vi "scan_DO_perform_scan.vi"(8 "error in (no error)":errorcluster, 10 "scan_settings":T1={"Center Pos. (mm)"=0.0, "Range [--|--]"=0.0, "Unit"=enum."mm", "Steps"=0.0, "Stage Number"=enum."1", "Stage Speed"=1.0, "Dwell Time (s)"=0.1, "Record Type"=enum."hdf5", "Save Path"=path "", "Notes"=""}, 11 "scan_panel in":refnum<class "scan_panel.lvclass">) -> (0 "error out":errorcluster, 3 "scan_panel out":refnum<class "scan_panel.lvclass">)   [LabVIEW 2015, in "scan_panel.lvclass"]
uses:
  scan_panel.lvclass
  scan_settings.ctl
  scan_unit.ctl
  scan_record.ctl
  scan_position_settings.ctl
  UI/front_panel_class/hardware_caller_queue_numbers.ctl
  Stage Class/Stage.lvclass
  Detector_Class/detector/detector.lvclass
  scan_hdf5_log/initialization_data.ctl
  scan_hdf5_log/scan_hdf5_log.lvclass
  Data Logger Class/data_logger.lvclass
  UI/panel_class/panel.lvclass
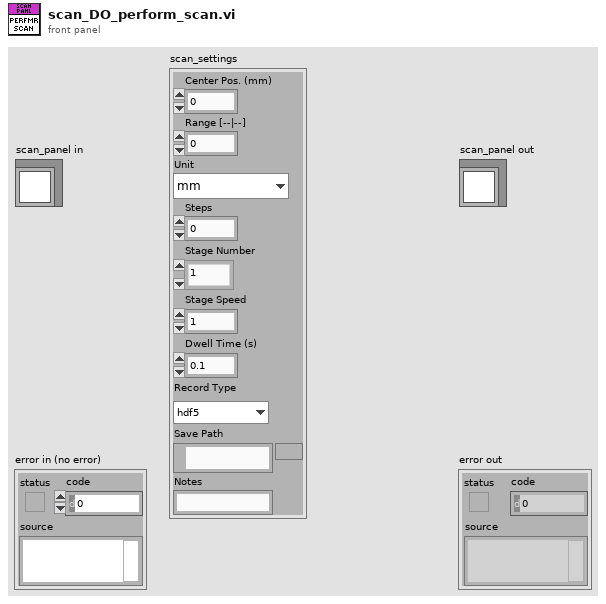
[diagram p1: front panel]
types:
  T1 = typedef "scan_settings.ctl" = cluster{"Center Pos. (mm)":dbl, "Range [--|--]":dbl, "Unit":T2, "Steps":dbl, "Stage Number":enum16{"1", "2"}, "Stage Speed":dbl, "Dwell Time (s)":dbl, "Record Type":T3, "Save Path":path, "Notes":string}
  T2 = typedef "scan_unit.ctl" = enum16{"mm", "s", "ms", "us", "ns", "ps", "fs"}
  T3 = typedef "scan_record.ctl" = enum16{"hdf5", "legacy", "None"}
  T4 = typedef "scan_position_settings.ctl" = cluster{"Center Pos. (mm)":dbl, "Range [--|--]":dbl, "Unit":T2, "Steps":dbl}
  T5 = typedef "initialization_data.ctl" = cluster{"Positions (mm)":dbl[], "dims":u32[]}
  T6 = typedef "hardware_caller_queue_numbers.ctl" = enum16{"stage1", "stage2", "experiment", "detector"}
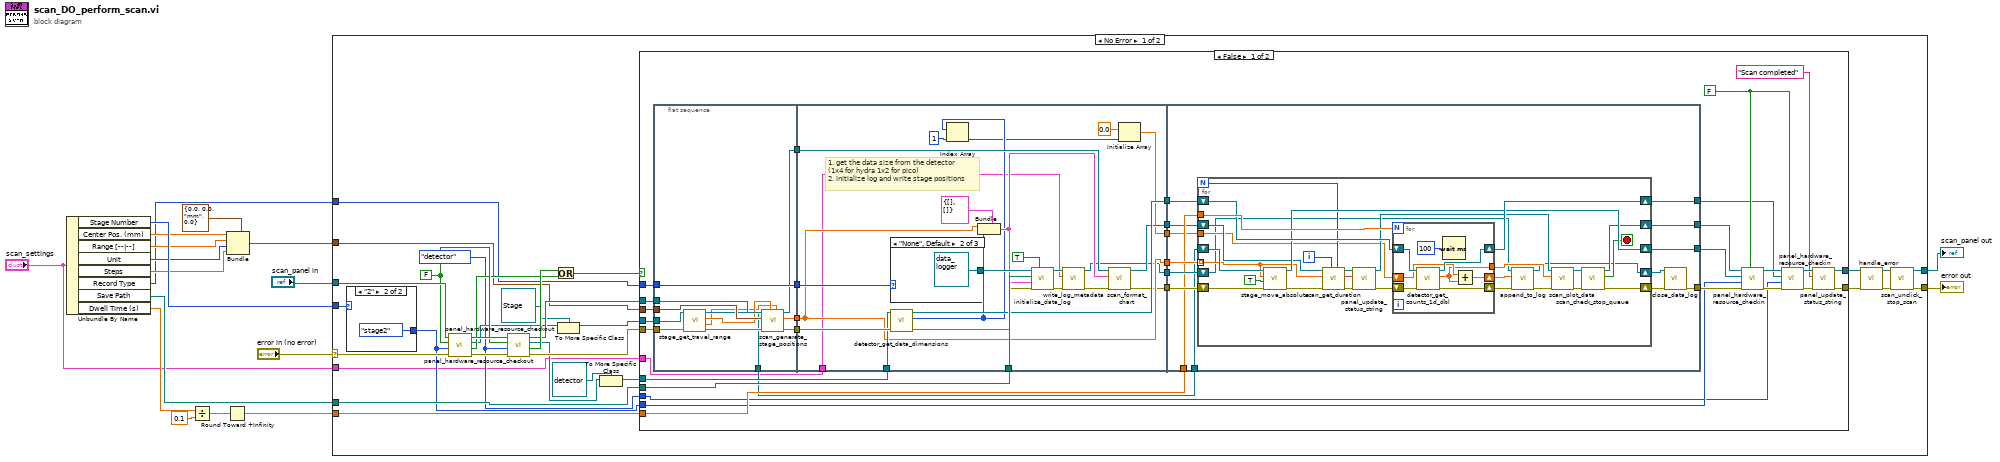
[diagram p0: block diagram]
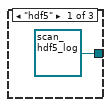
[diagram p2: hidden frame]
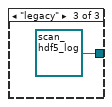
[diagram p3: hidden frame]
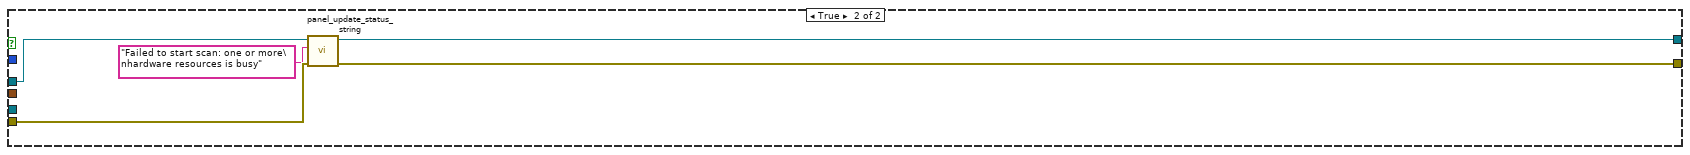
[diagram p4: hidden frame]
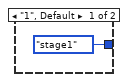
[diagram p5: hidden frame]
diagram:
  n1 = Unbundle By Name("scan_settings") -> ("Stage Number"=w14:enum16{"1", "2"}, "Center Pos. (mm)"=w13:dbl, "Range [--|--]"=w12:dbl, "Unit"=w11:T2, "Steps"=w10:dbl, "Record Type"=w7:T3, "Save Path"=w6:path, "Dwell Time (s)"=w5:dbl)
  n2 = Divide(x=w5, y=0.1) -> (x/y=w3:dbl)
  n3 = Round Toward +Infinity(x=w3) -> (ceil(x): smallest int >= x=w2:dbl)
  n4 = Bundle(cluster=T4 {"Center Pos. (mm)"=0.0, "Range [--|--]"=0.0, "Unit"=enum."mm", "Steps"=0.0} ("output cluster"), "Center Pos. (mm)"=w13, "Range [--|--]"=w12, "Unit"=w11, "Steps"=w10) -> (w8:T4)
  n5 = case shown="No Error" "error in (no error)" {
    selector: "error in (no error)" -> [w48 w181]
    tunnel: [w20 w181] -> w17
    tunnel: [w21 w180] -> w15
    tunnel: "scan_panel in" -> [w46 w180]
    tunnel: w14 -> [w47 _]
    tunnel: w8 -> [w37 _]
    tunnel: w7 -> [w36 _]
    tunnel: w6 -> [w35 _]
    tunnel: w2 -> [w28 _]
    tunnel: "scan_settings" -> [w19 _]
    frame No Error {
      w26 = hardware_caller_queue_numbers."detector" ("panel_number")
      w43 = FALSE ("Self?")
      n6 = case shown="\"2\"" w47 {
        tunnel: [hardware_caller_queue_numbers."stage1" ("panel_number") hardware_caller_queue_numbers."stage2" ("panel_number")] -> w27
        frame "1", Default {
        }
        frame "2" {
        }
      }
      n7 = call "panel_hardware_resource_checkout.vi"("error in (no error)"=w48, "panel_number"=w27, "Self?"=w43, "panel in"=w46) -> ("error out"=w45:errorcluster, "timed out?"=w41:bool, "hardware.lvclass"=w34:refnum<class "hardware.lvclass">, "panel out"=w44:refnum<class "scan_panel.lvclass">)  [unwired: 4 in]
      n8 = call "panel_hardware_resource_checkout.vi"("error in (no error)"=w45, "panel_number"=w26, "Self?"=w43, "panel in"=w44) -> ("error out"=w39:errorcluster, "timed out?"=w42:bool, "hardware.lvclass"=w31:refnum<class "hardware.lvclass">, "panel out"=w38:refnum<class "scan_panel.lvclass">)  [unwired: 4 in]
      n9 = Or(x=w42, y=w41) -> (x .or. y?=w40:bool)
      n10 = To More Specific Class(target class=refnum<class "Stage.lvclass"> refnum ("Stage.lvclass"), reference=w34) -> (specific class reference=w32:refnum<class "Stage.lvclass">)  [unwired: 1 in, 1 out]
      n11 = To More Specific Class(target class=refnum<class "detector.lvclass"> refnum ("detector.lvclass"), reference=w31) -> (specific class reference=w29:refnum<class "detector.lvclass">)  [unwired: 1 in, 1 out]
      n12 = case shown="False" w40 {
        tunnel: w39 -> [w79 w177]
        tunnel: w38 -> [w78 w175]
        tunnel: [w54 w174] -> w24
        tunnel: [w56 w176] -> w25
        tunnel: w37 -> [w77 _]
        tunnel: w36 -> [w75 _]
        tunnel: w35 -> [w73 _]
        tunnel: w32 -> [w51 _]
        tunnel: w29 -> [w70 _]
        tunnel: w28 -> [w64 _]
        tunnel: w27 -> [w61 _]
        tunnel: w26 -> [w59 _]
        tunnel: w19 -> [w49 _]
        frame False {
          w80 = FALSE ("Self")
          n13 = flat-sequence {
            tunnel: w79 -> [w88]
            tunnel: w78 -> [w94]
            tunnel: w77 -> [w93]
            tunnel: [w92] -> w76
            tunnel: w75 -> [w92]
            tunnel: [w91] -> w74
            tunnel: [w90] -> w72
            tunnel: [w89] -> w71
            tunnel: w51 -> [w86]
            tunnel: [w85] -> w50
            tunnel: w76 -> [w118]
            tunnel: w74 -> [w114]
            tunnel: w73 -> [w116]
            tunnel: w72 -> [w107]
            tunnel: w71 -> [w109]
            tunnel: w70 -> [w113]
            tunnel: [w106] -> w69
            tunnel: [w110] -> w68
            tunnel: [w97] -> w67
            tunnel: [w109] -> w66
            tunnel: [w108] -> w65
            tunnel: [w100] -> w52
            tunnel: w49 -> [w95]
            tunnel: w69 -> [w129]
            tunnel: w68 -> [w132]
            tunnel: w67 -> [w133]
            tunnel: w66 -> [w135]
            tunnel: w65 -> [w134]
            tunnel: w50 -> [w131]
            tunnel: w64 -> [w130]
            tunnel: [w126] -> w63
            tunnel: [w125] -> w62
            tunnel: [w124] -> w60
            tunnel: [w123] -> w58
            tunnel: w52 -> [w122]
            frame #0 {
              n14 = call-dynamic "stage_get_travel_range.vi"("error in (no error)"=w88, "Stage in"=w86) -> ("error out"=w87:errorcluster, "min(mm)"=w83:dbl, "max (mm)"=w84:dbl, "Stage out"=w85:refnum<class "Stage.lvclass">)  [unwired: 6 in]
              n15 = call "scan_generate_stage_positions.vi"("travel_min (mm)"=w83, "travel_max (mm)"=w84, "error in (no error)"=w87, "scan_position_settings"=w93, "scan_panel in"=w94) -> ("error out"=w91:errorcluster, "Positions (mm)"=w89:dbl[], "scan_panel out"=w90:refnum<class "scan_panel.lvclass">)  [unwired: 4 in]
            }
            frame #1 {
              # "1. get the data size from the detector \n(1x4 for hydra 1x2 for pico)\n2. initialize log and write stage positions"
              n16 = case shown="\"None\", Default" w118 {
                tunnel: [refnum<class "scan_hdf5_log.lvclass"> refnum ("scan_hdf5_log.lvclass") refnum<class "data_logger.lvclass"> refnum ("data_logger.lvclass") refnum<class "scan_hdf5_log.lvclass"> refnum ("scan_hdf5_log.lvclass")] -> w117
                frame "hdf5" {
                }
                frame "None", Default {
                }
                frame "legacy" {
                }
              }
              n17 = call-dynamic "detector_get_data_dimensions.vi"("error in (no error)"=w114, "detector in"=w113) -> ("error out"=w111:errorcluster, "dims"=w103:u32[], "detector out"=w110:refnum<class "detector.lvclass">)  [unwired: 6 in, 1 out]
              n18 = Index Array(array=w103, index=1) -> (element=w101:u32)
              n19 = Bundle(cluster=T5 {"Positions (mm)"=[], "dims"=[]} ("output cluster"), "Positions (mm)"=w109, "dims"=w103) -> (w105:T5)
              n20 = call-dynamic "initialize_data_log.vi"("Overwrite?"=TRUE, "error in (no error)"=w111, "Initialization Data"=w105, "Path"=w116, "data_logger in"=w117) -> ("error out"=w99:errorcluster, "data_logger out"=w98:refnum<class "data_logger.lvclass">)  [unwired: 5 in]
              n21 = call-dynamic "write_log_metadata.vi"("error in (no error)"=w99, "data"=w95, "data_logger in"=w98) -> ("error out"=w96:errorcluster, "data_logger out"=w97:refnum<class "data_logger.lvclass">)  [unwired: 7 in]
              n22 = call "scan_format_chart.vi"("error in (no error)"=w96, "info"=w105, "scan_panel in"=w107) -> ("error out"=w108:errorcluster, "panel out"=w106:refnum<class "scan_panel.lvclass">)  [unwired: 7 in]
              n23 = Initialize Array(0.0 ("element"), w101) -> (w100:dbl[])
            }
            frame #2 {
              n24 = for {
                N -> [w146]
                tunnel: w135 -> [w148] mode=indexing
                shift-right: [w157] -> w128
                shift-left: w134 -> [w161]
                shift-right: [w138] -> w127
                shift-left: w133 -> [w137]
                shift-right: [w162] -> w123
                shift-left: w132 -> [w163]
                shift-right: [w158] -> w124
                shift-left: w131 -> [w160]
                tunnel: w130 -> [w164]
                shift-right: [w156] -> w125
                shift-left: w129 -> [w152]
                tunnel: w122 -> [w141]
                i -> [w147]
                stop <- w155 stop-if-true
                n25 = call-dynamic "stage_move_absolute.vi"("error in (no error)"=w161, "wait_for_done"=TRUE, "Position"=w148, "Stage in"=w160) -> ("error out"=w153:errorcluster, "Stage out"=w158:refnum<class "Stage.lvclass">)  [unwired: 6 in]
                n26 = call "scan_get_duration.vi"("total_steps"=w146, "current_iteration"=w147, "error in (no error)"=w153, "current_position"=w148, "scan_panel in"=w152) -> ("error out"=w149:errorcluster, "time_remaining"=w150:string, "scan_panel out"=w151:refnum<class "scan_panel.lvclass">)  [unwired: 4 in]
                n27 = call-dynamic "panel_update_status_string.vi"("error in (no error)"=w149, "String"=w150, "scan_panel in"=w151) -> ("error out"=w154:errorcluster, "scan_panel out"=w144:refnum<class "scan_panel.lvclass">)  [unwired: 7 in]
                n28 = for {
                  N: w164 -> [_]
                  shift-right: [w170] -> w162
                  shift-left: w163 -> [w171]
                  shift-right: [w165] -> w140
                  shift-left: w154 -> [w169]
                  tunnel: [w167] -> w142
                  shift-right: [w166] -> w136
                  shift-left: w141 -> [w168]
                  n29 = call-dynamic "detector_get_counts_1d_dbl.vi"("error in (no error)"=w169, "detector in"=w171) -> ("error out"=w165:errorcluster, "counts"=w167:dbl[], "detector out"=w170:refnum<class "detector.lvclass">)  [unwired: 7 in]
                  n30 = Wait (ms)(milliseconds to wait=u32 100) -> ()  [unwired: 1 out]
                  n31 = Add(x=w168, y=w167) -> (x+y=w166:dbl[])
                }
                n32 = call-dynamic "append_to_log.vi"("error in (no error)"=w140, "Data"=w136, "data_logger in"=w137) -> ("error out"=w139:errorcluster, "data_logger out"=w138:refnum<class "data_logger.lvclass">)  [unwired: 7 in]
                n33 = call "scan_plot_data.vi"("error in (no error)"=w139, "data"=w142, "scan_panel in"=w144) -> ("error out"=w145:errorcluster, "scan_panel out"=w143:refnum<class "scan_panel.lvclass">)  [unwired: 7 in]
                n34 = call "scan_check_stop_queue.vi"("error in (no error)"=w145, "scan_panel in"=w143) -> ("error out"=w157:errorcluster, "stop?"=w155:bool, "scan_panel out"=w156:refnum<class "scan_panel.lvclass">)  [unwired: 7 in]
              }
              n35 = call-dynamic "close_data_log.vi"("error in (no error)"=w128, "data_logger in"=w127) -> ("error out"=w126:errorcluster)  [unwired: 8 in, 1 out]
            }
          }
          n36 = call "panel_hardware_resource_checkin.vi"("Self"=w80, "error in (no error)"=w63, "panel_number"=w61, "hardware.lvclass"=w60, "panel in"=w62) -> ("error out"=w82:errorcluster, "panel out"=w81:refnum<class "scan_panel.lvclass">)  [unwired: 5 in]
          n37 = call "panel_hardware_resource_checkin.vi"("Self"=w80, "error in (no error)"=w82, "panel_number"=w59, "hardware.lvclass"=w58, "panel in"=w81) -> ("error out"=w57:errorcluster, "panel out"=w55:refnum<class "scan_panel.lvclass">)  [unwired: 5 in]
          n38 = call-dynamic "panel_update_status_string.vi"("error in (no error)"=w57, "String"="Scan completed", "scan_panel in"=w55) -> ("error out"=w56:errorcluster, "scan_panel out"=w54:refnum<class "scan_panel.lvclass">)  [unwired: 7 in]
        }
        frame True {
          n39 = call-dynamic "panel_update_status_string.vi"("error in (no error)"=w177, "String"="Failed to start scan: one or more\nhardware resources is busy", "scan_panel in"=w175) -> ("error out"=w176:errorcluster, "scan_panel out"=w174:refnum<class "scan_panel.lvclass">)  [unwired: 7 in]
        }
      }
      n40 = call "handle_error.vi"("error in (no error)"=w25, "scan_panel in"=w24) -> ("error out"=w23:errorcluster, "scan_panel out"=w22:refnum<class "scan_panel.lvclass">)  [unwired: 8 in]
      n41 = call "scan_unclick_stop_scan.vi"("error in (no error)"=w23, "scan_panel in"=w22) -> ("error out"=w20:errorcluster, "scan_panel out"=w21:refnum<class "scan_panel.lvclass">)  [unwired: 8 in]
    }
    frame Error {
    }
  }
  "error out" <- w17
  "scan_panel out" <- w15
